vi "SVT Bearings.vi"   [LabVIEW 2017, in "SoundVib_MachineCharacteristic.lvlib"]
doc: "Calculates characteristic frequencies or orders of rolling-element bearings or hydrodynamic journal bearings. You must manually select the polymorphic instance you want to use."
uses:
  <vilib>/addons/Sound and Vibration/svt_Machine Characteristic/SoundVib_MachineCharacteristic.lvlib
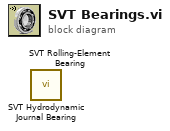
[diagram p0: block diagram]
diagram:
  n1 = call <vilib>:"SVT Hydrodynamic Journal Bearing.vi"() -> ()  [unwired: 14 in, 2 out]
  n2 = call <vilib>:"SVT Rolling-Element Bearing.vi"() -> ()  [unwired: 11 in, 5 out]
